vi "api_mqttPing.vi"(11 "error in (no error)":errorcluster) -> (4 "success":bool, 15 "error out":errorcluster)   [LabVIEW 2017, in "mqtt.lvclass"]
uses:
  mqtt.lvclass
  mqttTypedef/mqttRXdataCluster.ctl
  mqttTypedef/mqttFixedHeaderResponse.ctl
  mqttTypedef/mqttQOSlevel.ctl
  mqttTypedef/mqttMessageType.ctl
  mqttCmd/mqttCmdPing/mqttCmdPing.lvclass
  K:/Cutting Technology/1 - In scope projects/AI3568 Catapult Programme 2017-18/5 - Software Files/development/mqtt Folder/src/class/mqtt/mqttCmd/mqttCmd.lvclass
  mqttCmd/mqttCmd.lvclass/mqttCmd.ctl
  mqttCmd/mqttCmd.lvclass
panel:
  out "notification":T1
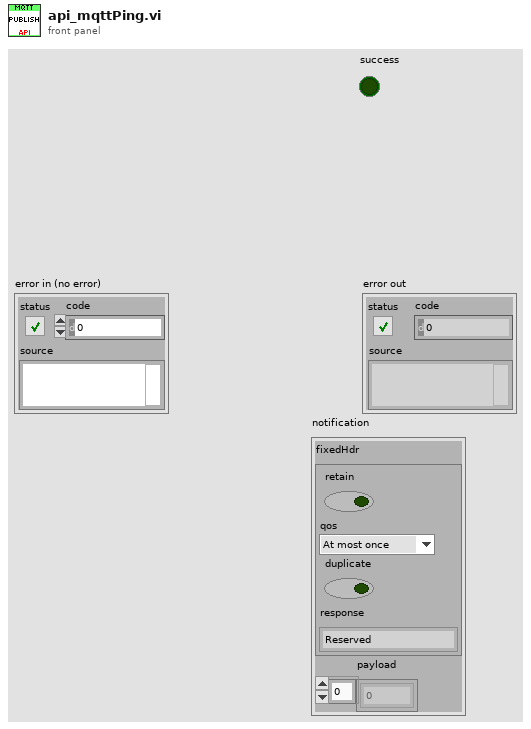
[diagram p1: front panel]
types:
  T1 = typedef "mqttRXdataCluster.ctl" = cluster{"fixedHdr":T2, "payload":u8[]}
  T2 = typedef "mqttFixedHeaderResponse.ctl" = cluster{"retain":bool, "qos":T3, "duplicate":bool, "response":T4}
  T3 = typedef "mqttQOSlevel.ctl" = enum8{"At most once", "At least once", "Exactly once", "Reserved"}
  T4 = typedef "mqttMessageType.ctl" = enum32{"Reserved", "CONNECT", "CONNACK", "PUBLISH", "PUBACK", "PUBREC", "PUBREL", "PUBCOMP", "SUBSCRIBE", "SUBACK", "UNSUBSCRIBE", "UNSUBACK", "PINGREQ", "PINGRESP", "DISCONNECT", "Reserved2"}
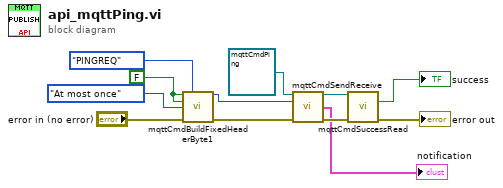
[diagram p0: block diagram]
diagram:
  w1 = FALSE ("retain(F)")
  n1 = call "mqttCmdBuildFixedHeaderByte1.vi"("retain(F)"=w1, "MessageType"=mqttMessageType."PINGREQ", "duplicate(F)"=w1, "QoS (At most once)"=mqttQOSlevel."At most once", "error in (no error)"="error in (no error)") -> ("byte1"=w2:u8, "error out"=w10:errorcluster)  [unwired: 9 in]
  n2 = call "mqttCmdSendReceive.vi"("mqttConnect in"=refnum<class "mqttCmdPing.lvclass"> refnum ("mqttCmdPing.lvclass"), "byte1"=w2, "error in (no error)"=w10) -> ("mqttConnect out"=w6:refnum<class "mqttCmdPing.lvclass">, "notification"=→"notification":T1, "error out"=w5:errorcluster)  [unwired: 10 in]
  n3 = call "mqttCmdSuccessRead.vi"("mqttBrokerCommand in"=w6, "error in (no error)"=w5) -> ("success"=→"success":bool, "error out"=→"error out":errorcluster)  [unwired: 11 in, 1 out]
